vi "drive inches.vi"(7 "inches to drive":dbl, 8 "error in (no error)":errorcluster, 11 "RobotDriveDevRef":T1={"DevStatus"={"status"=FALSE, "code"=0, "source"=""}, "Motors[]"=[], "Square Inputs"=FALSE, "Max Output"=1.0}) -> (0 "error out":errorcluster, 2 "done":bool, 3 "RobotDriveDevRef 2":T1={"DevStatus"={"status"=FALSE, "code"=0, "source"=""}, "Motors[]"=[], "Square Inputs"=FALSE, "Max Output"=1.0})   [LabVIEW 2016]
uses:
  <vilib>/Rock Robotics/WPI/RobotDrive/WPI_RobotDriveDevRef.ctl
  <vilib>/Rock Robotics/WPI/MotorControl/WPI_MotorControlDeviceRef.ctl
  <vilib>/Rock Robotics/WPI/MotorControl/WPI_MotorControlType.ctl
  <vilib>/Rock Robotics/SystemInterfaces/DIO/FPGA_DIOPWMChannel.ctl
  <vilib>/Rock Robotics/WPI/PWM/WPI_PWMDeadband.ctl
  Robot Global Data.vi
  <vilib>/Rock Robotics/WPI/RobotDrive/WPI_RobotDriveArcadeDrive_Standard(NoSaturation).vi
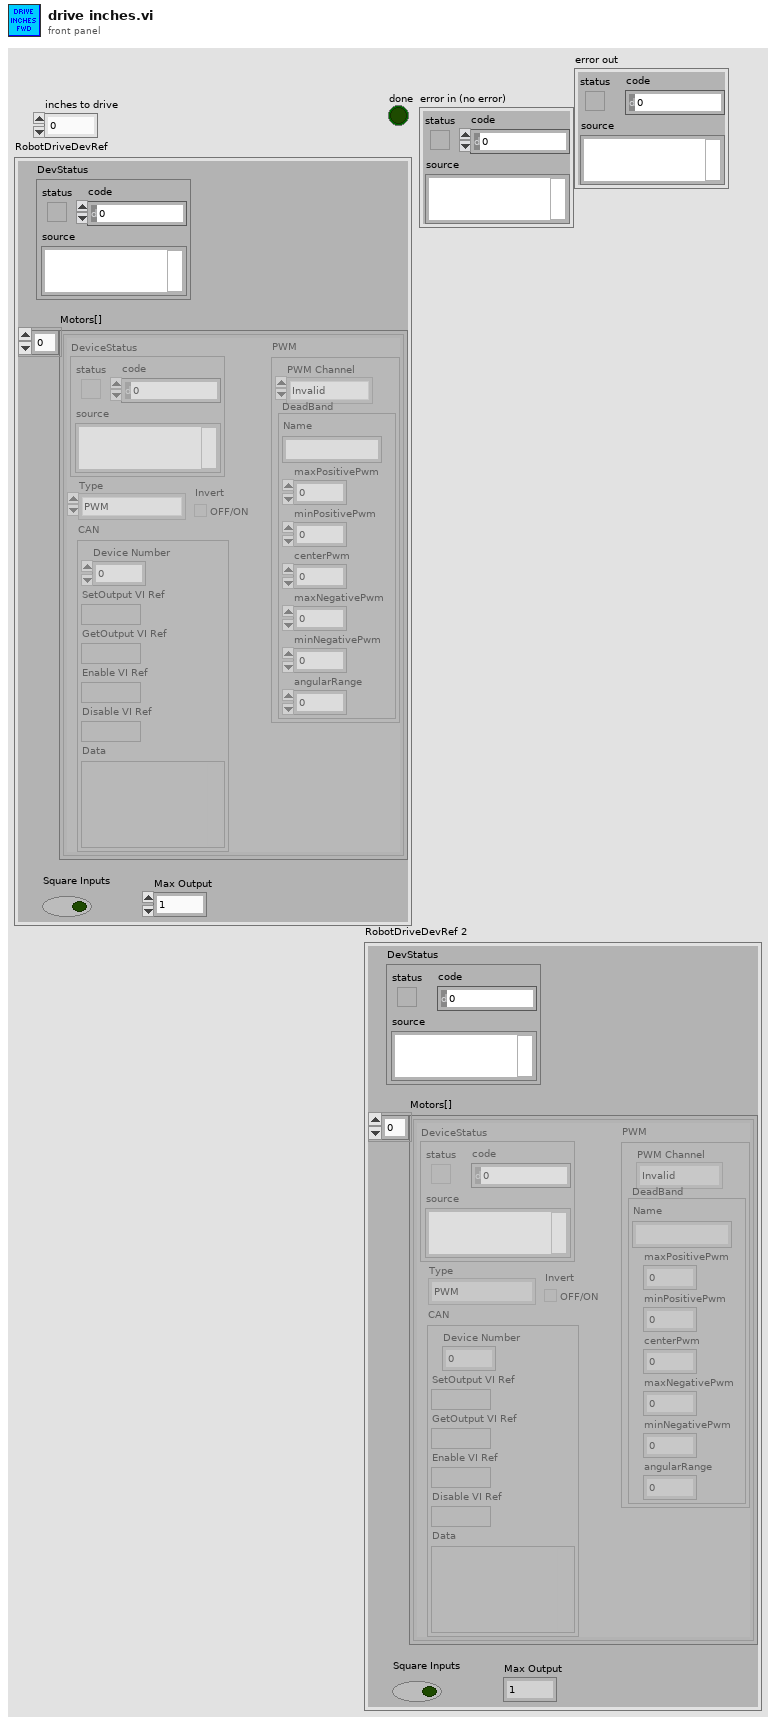
[diagram p1: front panel]
types:
  T1 = typedef "WPI_RobotDriveDevRef.ctl" = cluster{"DevStatus":errorcluster, "Motors[]":T2[], "Square Inputs":bool, "Max Output":dbl}
  T2 = typedef "WPI_MotorControlDeviceRef.ctl" = cluster{"DeviceStatus":errorcluster, "Type":T3, "PWM":cluster{"PWM Channel":T4, "DeadBand":T5}, "CAN":cluster{"Device Number":u8, "SetOutput VI Ref":variant, "GetOutput VI Ref":variant, "Enable VI Ref":variant, "Disable VI Ref":variant, "Data":variant}, "Invert":bool}
  T3 = typedef "WPI_MotorControlType.ctl" = enum16{"PWM", "CAN"}
  T4 = typedef "FPGA_DIOPWMChannel.ctl" = enum8{"PWM 0", "PWM 1", "PWM 2", "PWM 3", "PWM 4", "PWM 5", "PWM 6", "PWM 7", "PWM 8", "PWM 9", "PWM MXP 0", "PWM MXP 1", "PWM MXP 2", "PWM MXP 3", "PWM MXP 4", "PWM MXP 5", "PWM MXP 6", "PWM MXP 7", "PWM MXP 8", "PWM MXP 9", "Invalid"}
  T5 = typedef "WPI_PWMDeadband.ctl" = cluster{"Name":string, "maxPositivePwm":i32, "minPositivePwm":i32, "centerPwm":i32, "maxNegativePwm":i32, "minNegativePwm":i32, "angularRange":u16}
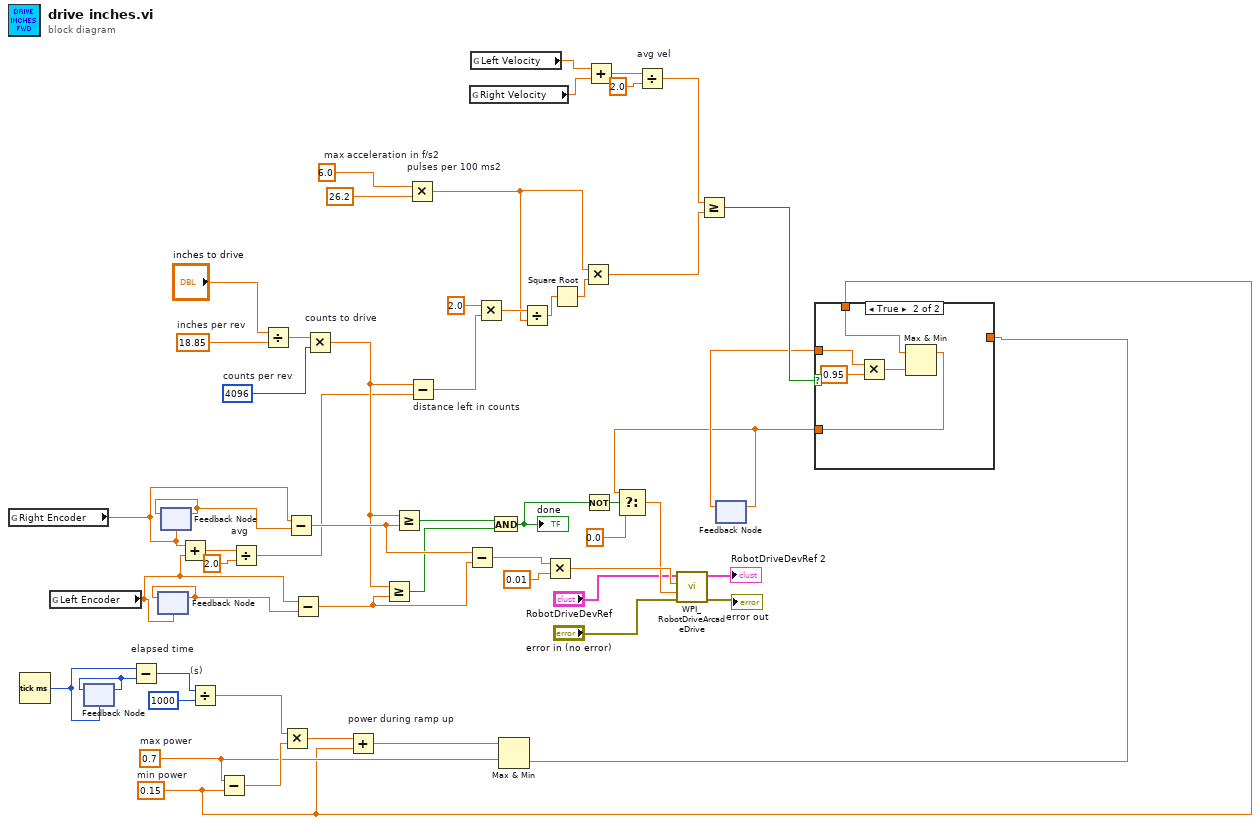
[diagram p0: block diagram]
diagram:
  w34 = 0.7  # max power
  w10 = 0.15  # min power
  w52 = 4096  # counts per rev
  w54 = 18.85  # inches per rev
  w33 = 6.0  # max acceleration in f/s2
  n1 = global read "Robot Global Data.vi" "Right Encoder"() -> (w31:dbl)
  n2 = Tick Count (ms)() -> (millisecond timer value=w41:u32)
  n3 = global read "Robot Global Data.vi" "Left Encoder"() -> (w30:dbl)
  n4 = feedback #1(w41) -> (w42:u32)
  n5 = feedback-in #1(w42) -> ()
  n6 = Subtract "elapsed time"(x=w41, y=w42) -> (x-y=w40:u32)
  n7 = feedback #2(w30) -> (w50:dbl)
  n8 = feedback-in #2(w50) -> ()
  n9 = feedback #3(w31) -> (w51:dbl)
  n10 = feedback-in #3(w51) -> ()
  n11 = Add(x=w31, y=w30) -> (x+y=w29:dbl)
  n12 = Divide "(s)"(x=w40, y=u32 1000) -> (x/y=w38:dbl)
  n13 = Subtract(x=w34, y=w10) -> (x-y=w35:dbl)
  n14 = Divide "avg"(x=w29, y=2.0) -> (x/y=w26:dbl)
  n15 = Divide(x="inches to drive", y=w54) -> (x/y=w53:dbl)
  n16 = Multiply(x=w38, y=w35) -> (x*y=w37:dbl)
  n17 = Subtract(x=w31, y=w51) -> (x-y=w49:dbl)
  n18 = Subtract(x=w30, y=w50) -> (x-y=w48:dbl)
  n19 = Multiply "counts to drive"(x=w53, y=w52) -> (x*y=w27:dbl)
  n20 = Add "power during ramp up"(x=w37, y=w10) -> (x+y=w36:dbl)
  n21 = Greater Or Equal?(x=w27, y=w48) -> (x >= y?=w44:bool)
  n22 = Greater Or Equal?(x=w27, y=w49) -> (x >= y?=w43:bool)
  n23 = Multiply "pulses per 100 ms2"(x=w33, y=26.2) -> (x*y=w20:dbl)
  n24 = Subtract "distance left in counts"(x=w27, y=w26) -> (x-y=w23:dbl)
  n25 = Subtract(x=w49, y=w48) -> (x-y=w47:dbl)
  n26 = global read "Robot Global Data.vi" "Right Velocity"() -> (w16:dbl)
  n27 = global read "Robot Global Data.vi" "Left Velocity"() -> (w17:dbl)
  n28 = Multiply(x=2.0, y=w23) -> (x*y=w22:dbl)
  n29 = And(x=w43, y=w44) -> (x .and. y?=w7:bool)
  "done" <- w7
  n30 = Max & Min(x=w36, y=w34) -> (min(x,y)=w12:dbl)  [unwired: 1 out]
  n31 = Divide(x=w22, y=w20) -> (x/y=w21:dbl)
  n32 = Multiply(x=w47, y=0.01) -> (x*y=w45:dbl)
  n33 = Square Root(x=w21) -> (sqrt(x)=w25:dbl)
  n34 = Multiply(x=w20, y=w25) -> (x*y=w14:dbl)
  n35 = Not(x=w7) -> (.not. x?=w6:bool)
  n36 = Add(x=w17, y=w16) -> (x+y=w18:dbl)
  n37 = Divide "avg vel"(x=w18, y=2.0) -> (x/y=w15:dbl)
  n38 = Greater Or Equal?(x=w15, y=w14) -> (x >= y?=w13:bool)
  n39 = feedback #4() -> (w11:dbl)  [unwired: 1 in]
  n40 = case shown="True" w13 {
    tunnel: w12 -> [w56 _]
    tunnel: [w56 w57] -> w9
    tunnel: w11 -> [_ w60]
    tunnel: w10 -> [_ w58]
    frame False {
    }
    frame True {
      n41 = Multiply(x=w60, y=0.95) -> (x*y=w59:dbl)
      n42 = Max & Min(x=w58, y=w59) -> (max(x,y)=w57:dbl)  [unwired: 1 out]
    }
  }
  n43 = Select(t=w9, s=w6, f=0.0) -> (s? t:f=w8:dbl)
  n44 = call-poly <vilib>:"WPI_RobotDriveArcadeDrive.vi"("error in (no error)"="error in (no error)", "Y axis value"=w8, "X axis value"=w45, "RobotDriveDevRef"="RobotDriveDevRef") -> ("error out"=→"error out":errorcluster, "RobotDriveDevRef"=→"RobotDriveDevRef 2":T1)  [unwired: 5 in, 1 out]
  n45 = feedback-in #4(w9) -> ()
